vi "set matrix.vi"(7 "m22":dbl, 8 "error in (no error)":errorcluster, 9 "m21":dbl, 10 "m12":dbl, 11 "m11":dbl) -> (0 "error out":errorcluster)   [LabVIEW 2015, in "SCANalone4x64.lvlib"]
doc: "__declspec(dllimport) void __stdcall set_matrix(double m11, double m12, double m21, double m22);"
uses:
  <userlib>/SCANalone4x64/SCANalone4x64.lvlib
  <userlib>/SCANalone4x64/SCANalone4x64.dll
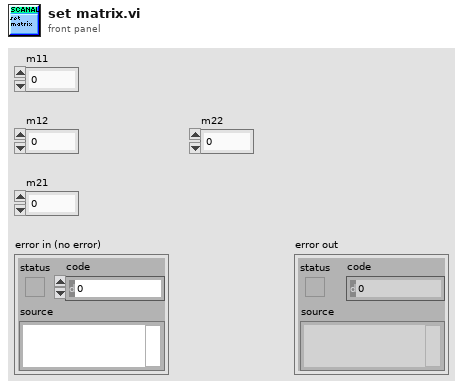
[diagram p1: front panel]
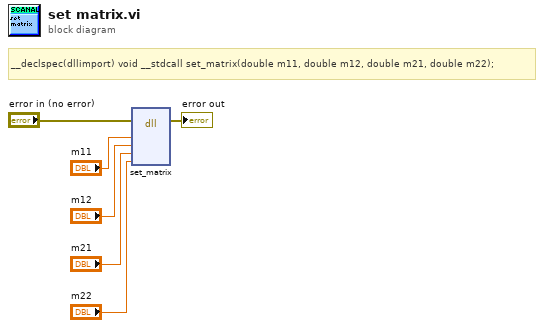
[diagram p0: block diagram]
diagram:
  # "__declspec(dllimport) void __stdcall set_matrix(double m11, double m12, double m21, double m22);"
  n1 = dll-call lib="C:/Program Files/National Instruments/LabVIEW 2015/user.lib/SCANalone4x64/SCANalone4x64.*" fn="set_matrix"(error in="error in (no error)", "m11"="m11", "m12"="m12", "m21"="m21", "m22"="m22") -> (error out=→"error out":errorcluster)  [unwired: 7 in, 1 out]
